vi "Write EQ data.vi"(8 "error in (no error)":errorcluster, 9 "gain correction (x/y)":dbl[](array[numeric]), 10 "frequency":dbl[](array[numeric]), 11 "file path":path) -> (0 "error out":errorcluster)   [LabVIEW 2022 SP3]
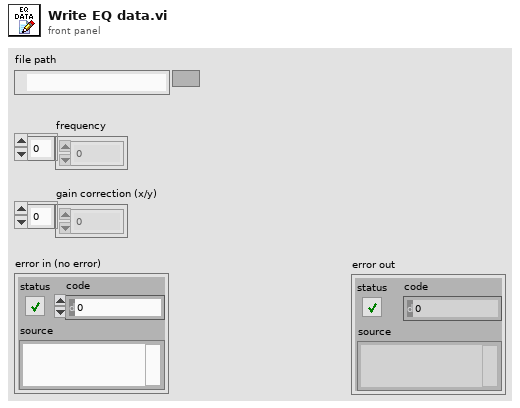
[diagram p1: front panel]
types:
  T1 = enum16{"open", "replace", "create", "open or create", "replace or create", "replace or create with confirmation"}
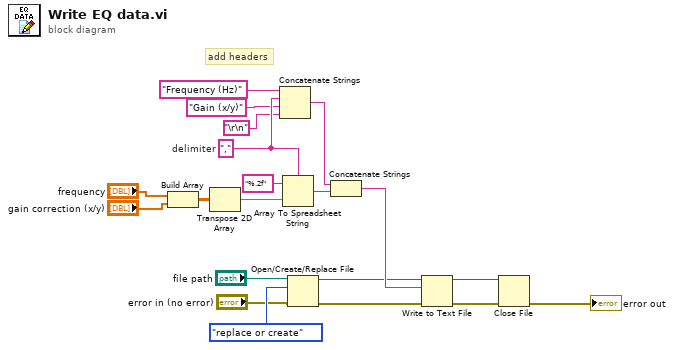
[diagram p0: block diagram]
diagram:
  w15 = ","  # delimiter
  # "add headers"
  n1 = Build Array("frequency", "gain correction (x/y)") -> (w17:dbl[][])
  n2 = Transpose 2D Array(2D array=w17) -> (transposed array=w16:dbl[][])
  n3 = Concatenate Strings("Frequency (Hz)" ("string"), w15, "Gain (x/y)" ("string"), "\r\n") -> (w11:string)
  n4 = Array To Spreadsheet String(delimiter (Tab)=w15, array=w16, 3:"%.2f" ("format string")) -> (spreadsheet string=w12:string)
  n5 = Open/Create/Replace File(file path (use dialog)="file path", error in="error in (no error)", operation (0:open)=T1."replace or create") -> (refnum out=w8:refnum<file>, error out=w7:errorcluster)  [unwired: 3 in, 1 out]
  n6 = Concatenate Strings(w11, w12) -> (w9:string)
  n7 = Write to Text File(file (use dialog)=w8, text=w9, error in=w7) -> (refnum out=w4:refnum<file>, error out=w5:errorcluster)  [unwired: 1 in, 1 out]
  n8 = Close File(refnum=w4, error in=w5) -> (error out=→"error out":errorcluster)  [unwired: 1 out]
